vi "InvokeCSComCollectNetGarbage.vi"(8 "error in (no error)":errorcluster) -> (0 "error out":errorcluster)   [LabVIEW 2017]
uses:
  C:/Code/CMCryoSysCode/Expose/COM/CSCom/CSCom/bin/Release/CSCom.dll
  COM/CSCom/CSCom/bin/Release/CSCom.dll
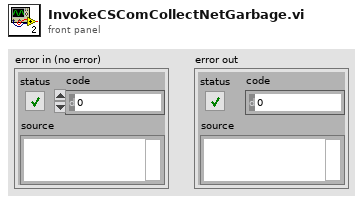
[diagram p1: front panel]
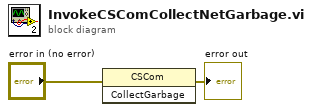
[diagram p0: block diagram]
diagram:
  n1 = invoke class="CSCom" method="CollectGarbage"(error in="error in (no error)") -> (error out=→"error out":errorcluster)  [unwired: 2 in, 2 out]
